vi "get_single_acq.vi"(8 "error in (no error)":errorcluster, 11 "stresing in":refnum<class "stresing.lvclass">) -> (0 "error out":errorcluster, 1 "trigger":dbl[][](array[numeric]), 2 "raw data":i32[][][](array[numeric]), 3 "stresing out":refnum<class "stresing.lvclass">)   [LabVIEW 2019, in "stresing.lvlib" / "stresing.lvclass"]
uses:
  stresing.lvclass
  D:/github/TransientAbsorptionDAQ.lv/_camera/_camera.lvlibp/_cameraClass/_camera.lvclass
  stresing.lvclass/stresing.ctl
  _camera/_camera.lvlibp/_cameraClass/Read background.vi
  driver/Stresing/board.vis/Globals.vi
  <vilib>/Analysis/NI_AALBase.lvlib
  <vilib>/Analysis/baseanly.llb/Mean (DBL).vi
panel:
  out "timing":u32
  out "size bg":i32
  out "size signal":i32
  out "Waveform Graph":i32[](graph)
  out "size(s) 3":i32[](array[numeric])
  out "size(s) 2":i32[](array[numeric])
  out "array w/ subset deleted 2":u16[][](array[numeric])
  out "array w/ subset deleted":u16[][](array[numeric])
  out "size(s)":i32[](array[numeric])
  out "deleted portion 2":u16[][](array[numeric])
  out "deleted portion":u16[][](array[numeric])
  # "1034-1088"
  # "0-9"
  # "10-1033"
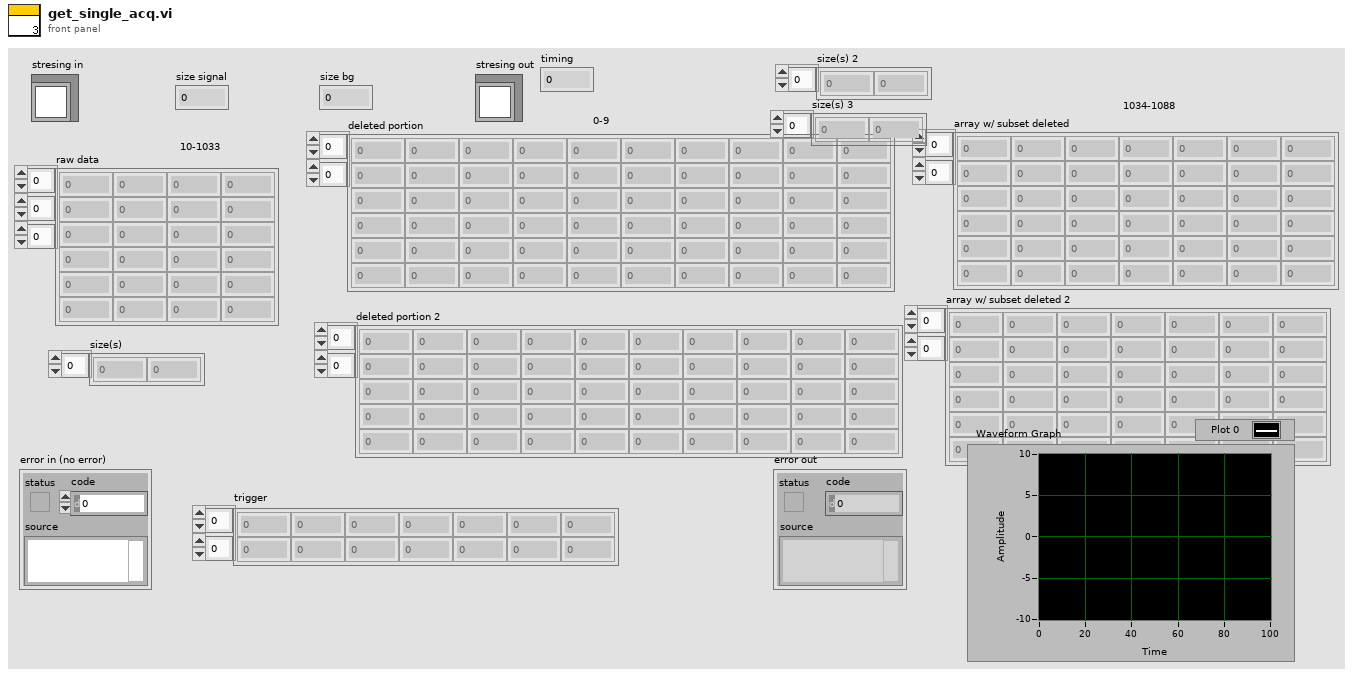
[diagram p1: front panel]
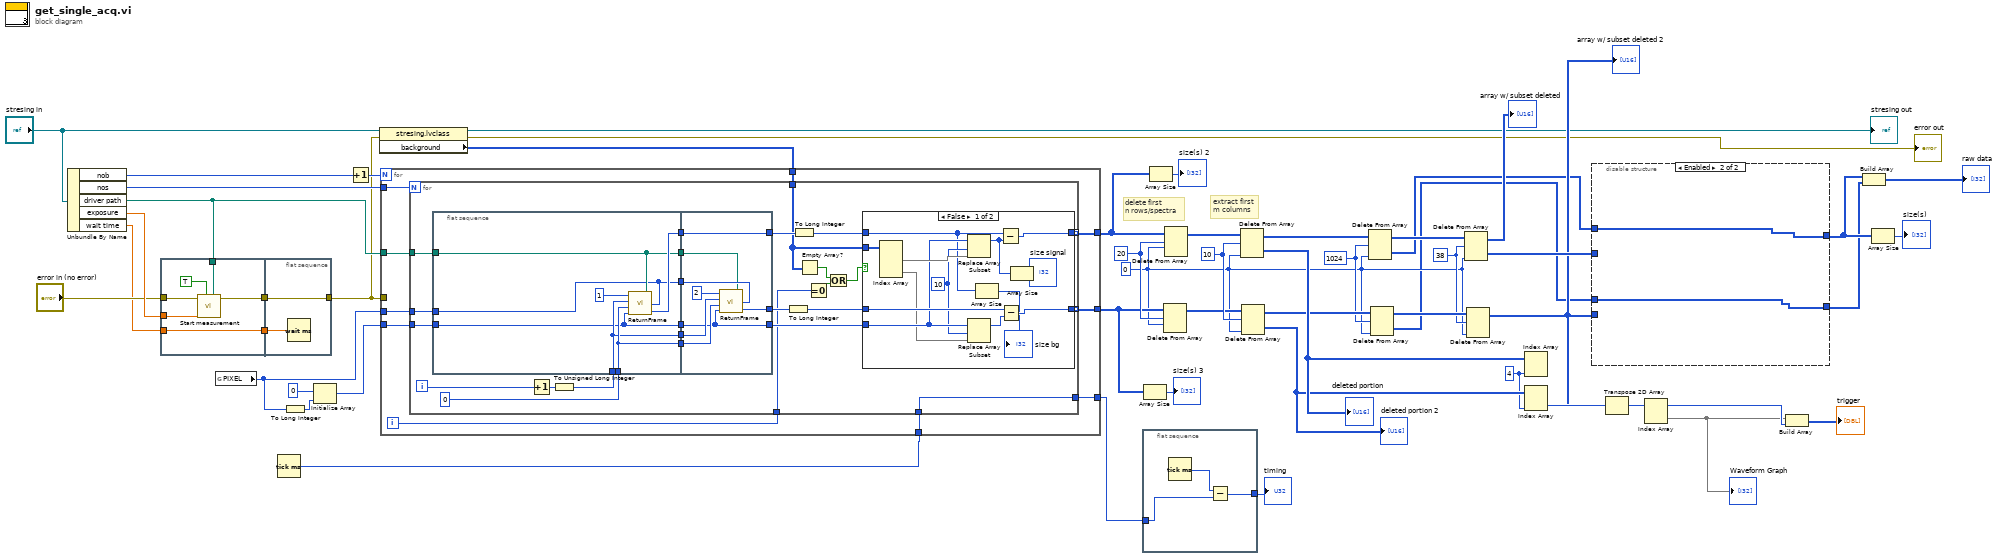
[diagram p0: block diagram]
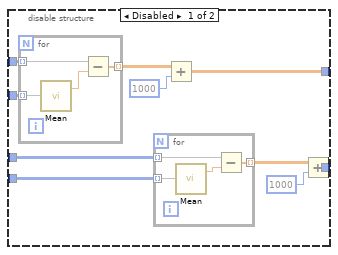
[diagram p2: hidden frame]
diagram:
  w22 = 38 ("length")
  w31 = 1024 ("length")
  w42 = 4 ("disabled index (col)")
  w47 = 10 ("length")
  w21 = 0 ("index (row)")
  w49 = 20 ("length")
  # "extract first\nm columns"
  # "delete first\nn rows/spectra"
  n1 = Unbundle By Name("stresing in") -> ("nob"=w51:u32, "nos"=w50:u32, "driver path"=w39:path, "exposure"=w38:dbl, "wait time"=w34:dbl)
  n2 = flat-sequence {
    tunnel: w39 -> [w58]
    tunnel: w38 -> [w56]
    tunnel: "error in (no error)" -> [w55]
    tunnel: [w54] -> w36
    tunnel: [w53] -> w35
    tunnel: w34 -> [w53]
    tunnel: [w60] -> w10
    tunnel: w36 -> [w60]
    tunnel: w35 -> [w59]
    frame #0 {
      n3 = call "Start measurement.vi"("driver path in"=w58, "extTrig"=TRUE, "Exposure"=w56, "Camera error in"=w55) -> ("Camera error out"=w54:errorcluster)  [unwired: 5 in]
    }
    frame #1 {
      n4 = Wait (ms)(milliseconds to wait=w59) -> ()  [unwired: 1 out]
    }
  }
  n5 = global read "Globals.vi" "PIXEL"() -> (w4:u32)
  n6 = Tick Count (ms)() -> (millisecond timer value=w3:u32)
  n7 = To Long Integer(number=w4) -> (32bit integer=w7:i32)
  n8 = Initialize Array(0, w7) -> (w5:i32[])
  n9 = Increment(x=w51) -> (x+1=w52:u32)
  n10 = property class="stresing.lvclass"(reference="stresing in", error in=w10) -> (reference out=→"stresing out":refnum<class "stresing.lvclass">, error out=→"error out":errorcluster, "background"=w8:i32[][])
  n11 = for {
    N: w52 -> [_]
    tunnel: w50 -> [w70]
    tunnel: [w69] -> w29
    tunnel: [w68] -> w26
    tunnel: w39 -> [w67]
    tunnel: w10 -> [_]
    tunnel: w8 -> [w66]
    tunnel: w5 -> [w65]
    tunnel: w4 -> [w64]
    tunnel: w3 -> [w62]
    tunnel: [w61] -> w2
    i -> [w63]
    n12 = for {
      N: w70 -> [_]
      tunnel: [w85] -> w69 mode=indexing
      tunnel: [w83] -> w68 mode=indexing
      tunnel: w67 -> [w87]
      tunnel: w66 -> [w81]
      tunnel: w65 -> [w77]
      tunnel: w64 -> [w76]
      tunnel: w63 -> [w73]
      tunnel: [w71] -> w61
      tunnel: w62 -> [w71]
      i -> [w94]
      n13 = flat-sequence {
        tunnel: [w112] -> w96
        tunnel: [w113] -> w95
        tunnel: w92 -> [w116]
        tunnel: u32 0 -> [w117]
        tunnel: [w117] -> w90
        tunnel: [w116] -> w89
        tunnel: [w115] -> w88
        tunnel: w87 -> [w114]
        tunnel: [w114] -> w86
        tunnel: w77 -> [w113]
        tunnel: w76 -> [w112]
        tunnel: w96 -> [w125]
        tunnel: w95 -> [w119]
        tunnel: w90 -> [w124]
        tunnel: w89 -> [w123]
        tunnel: [w122] -> w84
        tunnel: w88 -> [w122]
        tunnel: [w121] -> w82
        tunnel: w86 -> [w120]
        tunnel: [w119] -> w80
        frame #0 {
          n14 = call "ReturnFrame.vi"("length"=w112, "path in"=w114, "Data Values In"=w113, "curr_nob"=w117, "curr_nos"=w116, "Drv"=u32 1) -> ("Data Values Out"=w115:u16[])
        }
        frame #1 {
          n15 = call "ReturnFrame.vi"("length"=w125, "path in"=w120, "Data Values In"=w119, "curr_nob"=w124, "curr_nos"=w123, "Drv"=u32 2) -> ("Data Values Out"=w121:u16[])
        }
      }
      n16 = Increment(x=w94) -> (x+1=w93:i32)
      n17 = To Unsigned Long Integer(number=w93) -> (unsigned 32bit integer=w92:u32)
      n18 = To Long Integer(number=w82) -> (32bit integer=w78:i32[])
      n19 = To Long Integer(number=w84) -> (32bit integer=w79:i32[])
      n20 = Empty Array?(array=w81) -> (empty?=w75:bool)
      n21 = Equal To 0?(x=w73) -> (x = 0?=w74:bool)
      n22 = Or(x=w75, y=w74) -> (x .or. y?=w72:bool)
      n23 = case shown="False" w72 {
        tunnel: [w108 w111] -> w85
        tunnel: w79 -> [w98 w111]
        tunnel: [w106 w110] -> w83
        tunnel: w78 -> [w107 w110]
        tunnel: w81 -> [w109 _]
        tunnel: w80 -> [w104 _]
        frame False {
          w103 = 10 ("index")
          n24 = Index Array(array=w109) -> (element #1=w105:i32[], element #2=w102:i32[])  [unwired: 4 in]
          n25 = Replace Array Subset(array=w104, new element=w105, index=w103) -> (w100:i32[])
          n26 = Replace Array Subset(array=w104, new element=w102, index=w103) -> (w101:i32[])
          n27 = Array Size(array=w98) -> (size(s)=→"size bg":i32)
          n28 = Subtract(x=w98, y=w100) -> (x-y=w108:i32[])
          n29 = Subtract(x=w107, y=w101) -> (x-y=w106:i32[])
          n30 = Array Size(array=w100) -> (size(s)=→"size signal":i32)
        }
        frame True {
        }
      }
    }
  }
  n31 = flat-sequence {
    tunnel: w2 -> [w128]
    tunnel: [w127] -> w1
    frame #0 {
      n32 = Tick Count (ms)() -> (millisecond timer value=w129:u32)
      n33 = Subtract(x=w129, y=w128) -> (x-y=w127:u32)
    }
  }
  n34 = Array Size(array=w26) -> (size(s)=→"size(s) 3":i32[])
  n35 = Array Size(array=w29) -> (size(s)=→"size(s) 2":i32[])
  n36 = Delete From Array(array=w26, length=w49, index (row)=w21) -> (array with subset deleted=w46:i32[][])  [unwired: 1 in, 1 out]
  n37 = Delete From Array(array=w29, length=w49, index (row)=w21) -> (array with subset deleted=w48:i32[][])  [unwired: 1 in, 1 out]
  n38 = Delete From Array(array=w48, length=w47, index (col)=w21) -> (deleted portion=w44:i32[][], array with subset deleted=w33:i32[][])  [unwired: 1 in]
  "deleted portion" <- w44
  n39 = Delete From Array(array=w46, length=w47, index (col)=w21) -> (deleted portion=w43:i32[][], array with subset deleted=w32:i32[][])  [unwired: 1 in]
  "deleted portion 2" <- w43
  n40 = Delete From Array(array=w33, length=w31, index (col)=w21) -> (deleted portion=w16:i32[][], array with subset deleted=w25:i32[][])  [unwired: 1 in]
  n41 = Delete From Array(array=w32, length=w31, index (col)=w21) -> (deleted portion=w14:i32[][], array with subset deleted=w23:i32[][])  [unwired: 1 in]
  n42 = Delete From Array(array=w25, length=w22, index (col)=w21) -> (deleted portion=w18:i32[][], array with subset deleted=→"array w/ subset deleted":i32[][])  [unwired: 1 in]
  n43 = Delete From Array(array=w23, length=w22, index (col)=w21) -> (array with subset deleted=w17:i32[][])  [unwired: 1 in, 1 out]
  "array w/ subset deleted 2" <- w17
  n44 = Index Array(array=w44, index (col)=w42) -> ()  [unwired: 1 in, 1 out]
  n45 = Index Array(array=w43, index (col)=w42) -> (element=w41:i32[])  [unwired: 1 in]
  n46 = disable-structure shown="Enabled" {
    disable-tunnel: w18 -> [w139 _]
    disable-tunnel: w17 -> [w138 _]
    disable-tunnel: w16 -> [w137 w149]
    disable-tunnel: [w134 w149] -> w15
    disable-tunnel: w14 -> [w133 w148]
    disable-tunnel: [w130 w148] -> w13
    frame Disabled {
      n47 = for {
        tunnel: w139 -> [w147] mode=indexing
        tunnel: w137 -> [w146] mode=indexing
        tunnel: [w144] -> w136 mode=indexing
        n48 = call-poly <vilib>:"Mean.vi"("X"=w147) -> ("mean"=w145:dbl)  [unwired: 1 out]
        n49 = Subtract(x=w146, y=w145) -> (x-y=w144:dbl[])
      }
      n50 = for {
        tunnel: w138 -> [w143] mode=indexing
        tunnel: w133 -> [w142] mode=indexing
        tunnel: [w140] -> w131 mode=indexing
        n51 = call-poly <vilib>:"Mean.vi"("X"=w143) -> ("mean"=w141:dbl)  [unwired: 1 out]
        n52 = Subtract(x=w142, y=w141) -> (x-y=w140:dbl[])
      }
      n53 = Add(x=w136, y=1000) -> (x+y=w134:dbl[][])
      n54 = Add(x=w131, y=1000) -> (x+y=w130:dbl[][])
    }
    frame Enabled {
    }
  }
  n55 = Transpose 2D Array(2D array=w17) -> (transposed array=w19:i32[][])
  n56 = Index Array(array=w19) -> (element=w20:i32[])  [unwired: 2 in]
  "Waveform Graph" <- w20
  n57 = Build Array(w20, w41) -> (→"trigger":i32[][])
  n58 = Build Array(w15, w13) -> (→"raw data":i32[][][])
  n59 = Array Size(array=w15) -> (size(s)=→"size(s)":i32[])
  "timing" <- w1
